vi "SEARCH_volumes.vi"(8 "error in (no error)":errorcluster, 11 "REST Client in":refnum<class "REST Client.lvclass">) -> (3 "REST Client out":refnum<class "REST Client.lvclass">)   [LabVIEW 2024, in "CV_RESTful_Lib.lvlib"]
uses:
  CV_RESTful_Lib.lvlib
  <vilib>/addons/_JKI.lib/REST Client/classes/REST Client/REST Client.lvclass
  typedefs/cv_volume.search--cluster.ctl
  typedefs/cv_volume.search.results--cluster.ctl
  typedefs/cv_volume.issue--cluster.ctl
  typedefs/cv_volume.publisher--cluster.ctl
  <vilib>/addons/_JKI.lib/REST Client/classes/REST Client/HTTP Header.ctl
  <vilib>/NI/Advanced HTTP Client/Header--Combo Box.ctl
  <vilib>/NI/Advanced HTTP Client/Session.lvclass
  <vilib>/addons/_JKI.lib/Serialization/JSON/JKI JSON Serialization.lvlib
panel:
  out "size(s)":i32
  out "resulting string":string
  in  "offset":i32
  in  "search string":string="Avengers"
  out "search results":T1
  out "error out":errorcluster
  out "Status String":string
  out "Status Code":u16
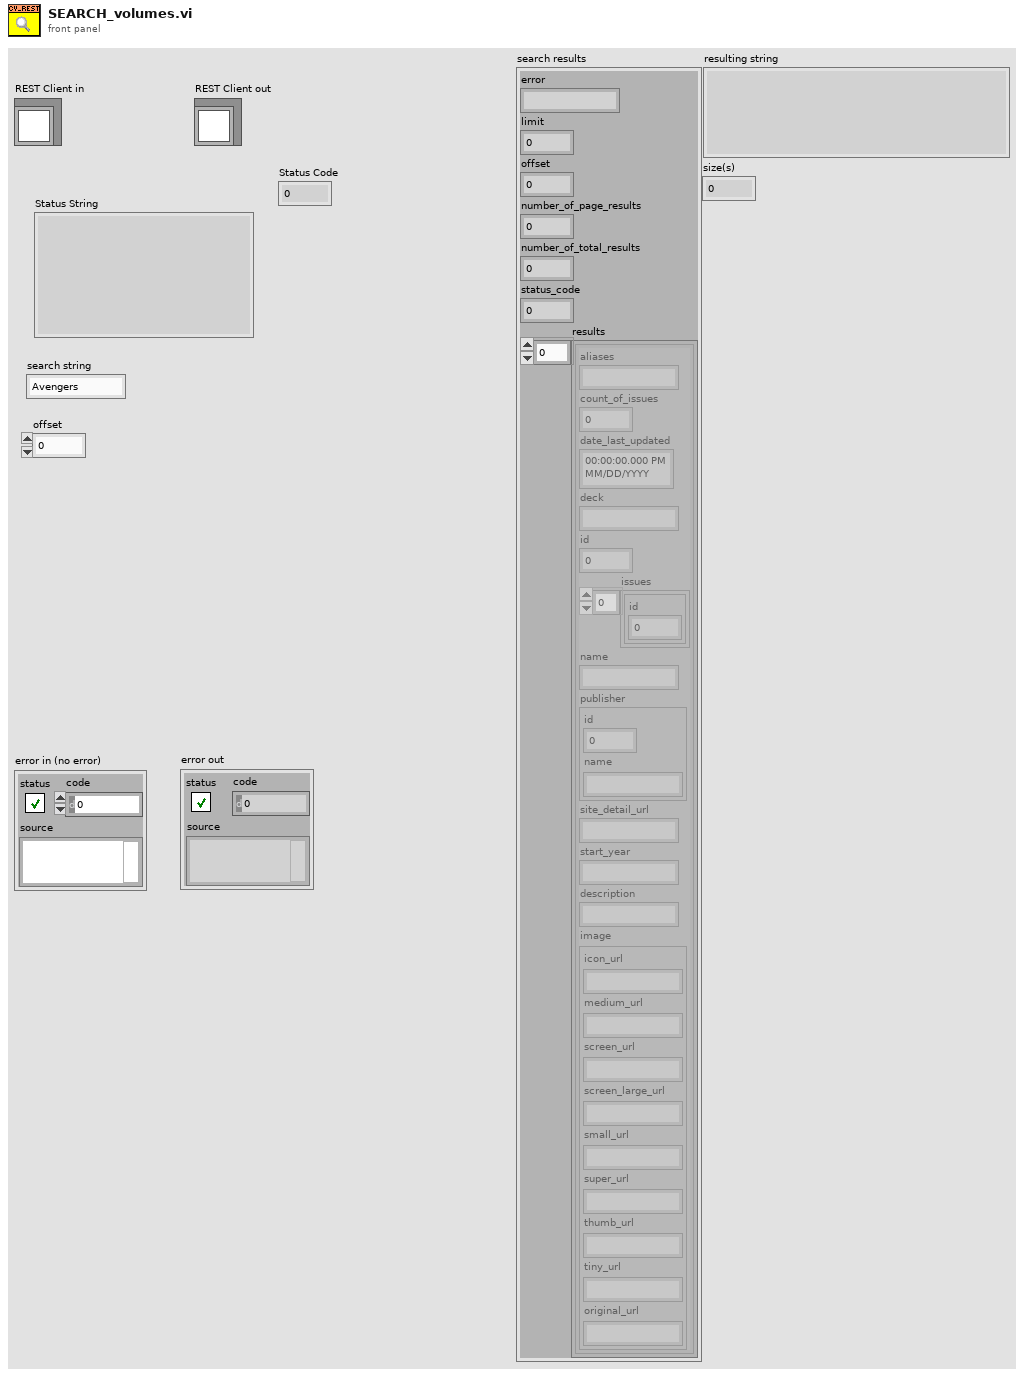
[diagram p1: front panel]
types:
  T1 = typedef "CV_RESTful_Lib.lvlib/cv_volume.search--cluster.ctl" = cluster{"error":string, "limit":i32, "offset":i32, "number_of_page_results":i32, "number_of_total_results":i32, "status_code":i32, "results":T2}
  T2 = typedef "CV_RESTful_Lib.lvlib/cv_volume.search.results--cluster.ctl" = cluster{"aliases":string, "count_of_issues":i32, "date_last_updated":timestamp, "deck":string, "id":i32, "issues":T3[], "name":string, "publisher":T4, "site_detail_url":string, "start_year":string, "description":string, "image":cluster{"icon_url":string, "medium_url":string, "screen_url":string, "screen_large_url":string, "small_url":string, "super_url":string, "thumb_url":string, "tiny_url":string, "original_url":string}}[]
  T3 = typedef "CV_RESTful_Lib.lvlib/cv_volume.issue--cluster.ctl" = cluster{"id":i32}
  T4 = typedef "CV_RESTful_Lib.lvlib/cv_volume.publisher--cluster.ctl" = cluster{"id":i32, "name":string}
  T5 = typedef "REST Client.lvlib/REST Client.lvclass/HTTP Header.ctl" = cluster{"header":T6, "value":string}
  T6 = typedef "lib_NI_Advanced HTTP Client.lvlib/Session.lvclass/Header--Combo Box.ctl" = string
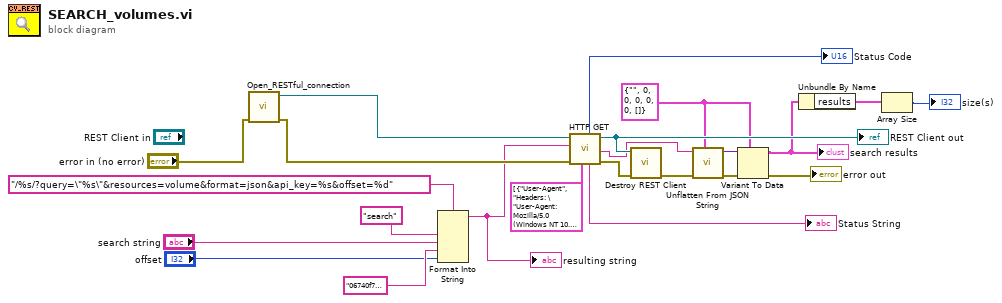
[diagram p0: block diagram]
diagram:
  w9 = T1 {"error"="", "limit"=0, "offset"=0, "number_of_page_results"=0, "number_of_total_results"=0, "status_code"=0, "results"=[]} ("volume")
  n1 = call "Open_RESTful_connection.vi"("error in (no error)"="error in (no error)") -> ("error out"=w16:errorcluster, "REST Client out"=w15:refnum<class "REST Client.lvclass">)  [unwired: 9 in]
  n2 = Format Into String(format string="/%s/?query=\"%s\"&resources=volume&format=json&api_key=%s&offset=%d", "search" ("resource"), "search string", "06740f73403e0b211d597c50ea94c7f16ea5e8ea", "offset") -> (resulting string=w6:string)  [unwired: 2 in, 1 out]
  "resulting string" <- w6
  n3 = call-dynamic "HTTP GET.vi"("request specific headers"=T5[] [{"header"="User-Agent", "value"="Headers: \"User-Agent: Mozilla/5.0 (Windows NT 10.0; Win64; x64) AppleWebKit/537.36 (KHTML, like Gecko) Chrome/91.0.4472.101 Safari/537.36\""}], "error in (no error)"=w16, "Path"=w6, "REST Client in"=w15) -> ("error out"=w13:errorcluster, "Response body"=w10:string, "REST Client out"=w14:refnum<class "REST Client.lvclass">, "Status String"=→"Status String":string, "Status Code"=→"Status Code":u16)  [unwired: 2 in, 1 out]
  "REST Client out" <- w14
  n4 = call-dynamic "Destroy REST Client.vi"("error in (no error)"=w13, "REST Client in"=w14) -> ("error out"=w12:errorcluster)  [unwired: 9 in]
  n5 = call <vilib>:"Unflatten From JSON String.vi"("Type and Defaults"=w9, "error in"=w12, "JSON String"=w10) -> ("error out"=w11:errorcluster, "Variant"=w8:variant)  [unwired: 7 in]
  n6 = Variant To Data(error in=w11, type=w9, Variant=w8) -> (data=w3:T1, error out=→"error out":errorcluster)
  "search results" <- w3
  n7 = Unbundle By Name(w3) -> ("results"=w2:T2)
  n8 = Array Size(array=w2) -> (size(s)=→"size(s)":i32)
